vi "SaveImagesFromArray (SubVI).vi"(8 "error in (no error)":errorcluster, 9 "Array of Images":T1[](array[typedef]), 10 "XY Camera Coordinates":dbl[][](array[numeric]), 11 "Path to save collected images":path=path "E:/XYZstage+Camera_CollectedImages/12-17-2016/images") -> (0 "error out":errorcluster)   [LabVIEW 2016]
uses:
  <vilib>/vision/Image Controls.llb/IMAQ Image.ctl
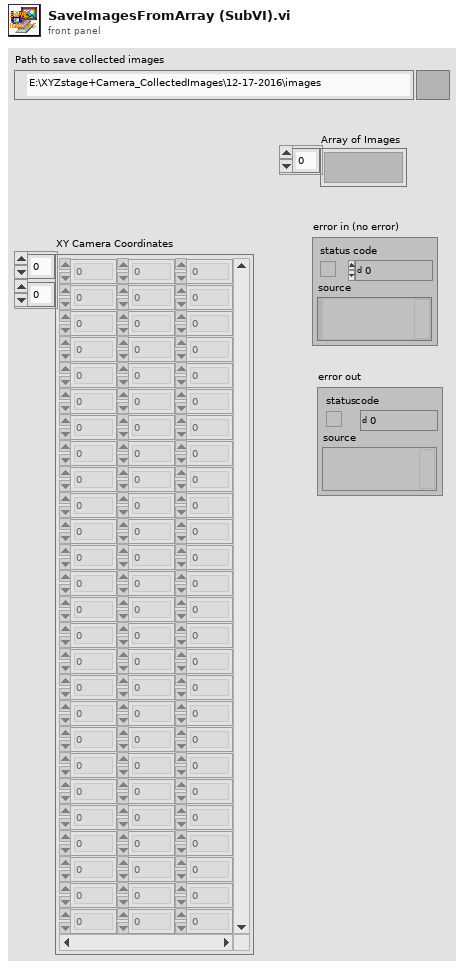
[diagram p1: front panel]
types:
  T1 = typedef "IMAQ Image.ctl" = refnum<image>
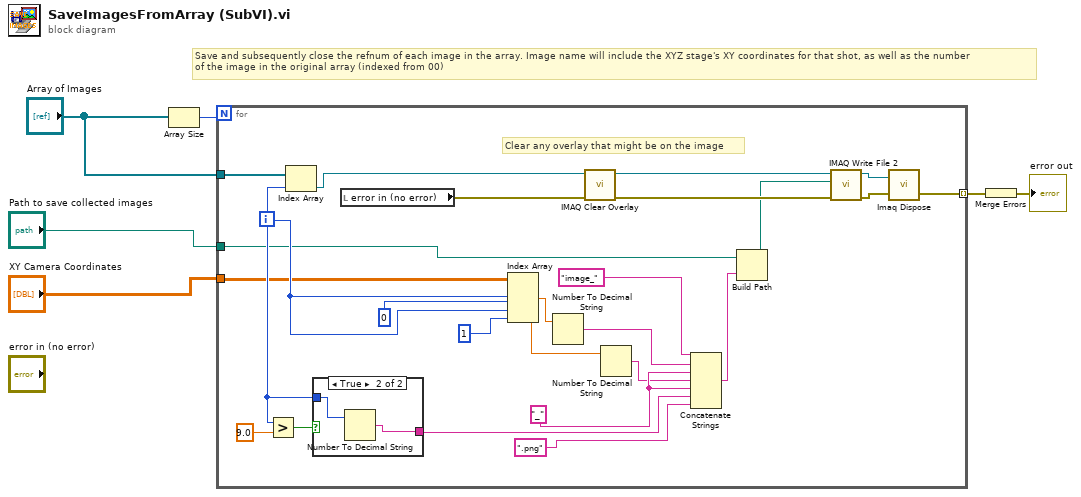
[diagram p0: block diagram]
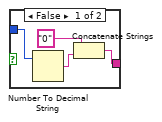
[diagram p2: hidden frame]
diagram:
  # "Save and subsequently close the refnum of each image in the array. Image name will include the XYZ stage's XY coordinates for that shot, as well as the number\nof the image in the original array (indexed from 00)"
  n1 = Array Size(array="Array of Images") -> (size(s)=w3:i32)
  n2 = for {
    N: w3 -> [_]
    tunnel: "Array of Images" -> [w31]
    tunnel: "Path to save collected images" -> [w16]
    tunnel: "XY Camera Coordinates" -> [w15]
    tunnel: [w12] -> w2 mode=indexing
    i -> [w17]
    w20 = "_" ("string")
    # "Clear any overlay that might be on the image"
    n3 = Greater?(x=w17, y=9.0) -> (0:w29:bool)
    n4 = Index Array(array=w31, index=w17) -> (element=w11:T1)
    n5 = case shown="True" w29 {
      tunnel: w17 -> [w35 w37]
      tunnel: [w32 w36] -> w26
      frame False {
        n6 = Number To Decimal String(number=w35) -> (decimal integer string=w34:string)  [unwired: 1 in]
        n7 = Concatenate Strings("0" ("string"), w34) -> (w32:string)
      }
      frame True {
        n8 = Number To Decimal String(number=w37) -> (decimal integer string=w36:string)  [unwired: 1 in]
      }
    }
    n9 = local read "error in (no error)"() -> (w10:errorcluster)
    n10 = Index Array(array=w15, index (row) #1=w17, index (col) #1=0 ("disabled index (col)"), index (row) #2=w17, index (col) #2=1 ("disabled index (col)")) -> (element #1=w23:dbl, element #2=w18:dbl)
    n11 = Number To Decimal String(number=w23) -> (decimal integer string=w21:string)  [unwired: 1 in]
    n12 = call "IMAQ Clear Overlay"("error in (no error)"=w10, "Image"=w11) -> ("error out"=w9:errorcluster, "Image Out"=w8:T1)  [unwired: 8 in]
    n13 = Number To Decimal String(number=w18) -> (decimal integer string=w19:string)  [unwired: 1 in]
    n14 = Concatenate Strings("image_" ("string"), w21, w20, w19, w20, w26, ".png" ("string")) -> (w28:string)
    n15 = Build Path(base path=w16, name or relative path=w28) -> (appended path=w7:path)
    n16 = call-poly "IMAQ Write File 2"("error in (no error)"=w9, "File Path"=w7, "Image"=w8) -> ("error out"=w13:errorcluster, "Image Out (duplicate)"=w14:T1)  [unwired: 7 in]
    n17 = call "Imaq Dispose"("Image"=w14, "error in (no error)"=w13) -> ("error out"=w12:errorcluster)  [unwired: 4 in]
  }
  n18 = Merge Errors(w2) -> (→"error out":errorcluster)
